vi "LinxUartGetBytesAvailable.vi"(8 "Error In":errorcluster, 10 "Uart Channel":u8, 11 "LINX Resource":T1) -> (0 "Error Out":errorcluster, 1 "Num Bytes":u8, 3 "LINX Resource":T1)   [LabVIEW 2011, in "LMH-LINX.lvlib" / "Local IO.lvlib"]
uses:
  Local IO.lvlib
  Type Defs/LINX Ref.ctl
  Type Defs/Platform.ctl
  Type Defs/Interface.ctl
  Device/Type Defs/LINX Device Config.ctl
  Device/Type Defs/TCP Config.ctl
  Device/Type Defs/Channels.ctl
  Type Defs/Error Type.ctl
  LMH-LINX.lvlib
  Type Defs/Channel FGV States.ctl
  liblinxdevice.dll
  Device/Device.lvlib
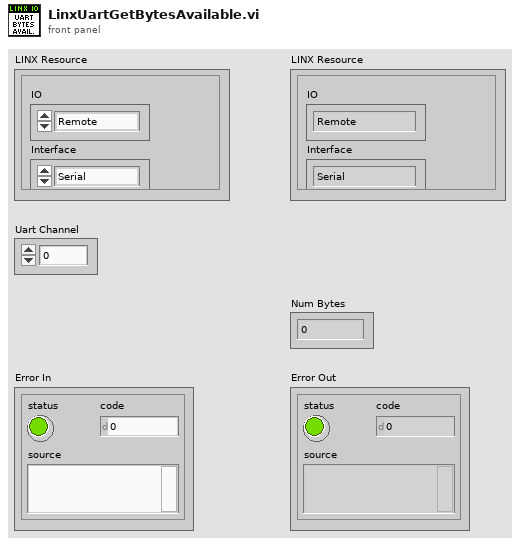
[diagram p1: front panel]
types:
  T1 = typedef "LMH-LINX.lvlib/LINX Ref.ctl" = cluster{"IO":T2, "Interface":T3, "LINX Device Config":T4}
  T2 = typedef "LMH-LINX.lvlib/Platform.ctl" = enum16{"Remote", "Local"}
  T3 = typedef "LMH-LINX.lvlib/Interface.ctl" = enum16{"Serial", "TCP"}
  T4 = typedef "LMH-LINX.lvlib/Device.lvlib/LINX Device Config.ctl" = cluster{"Interface":T3, "COM Port":refnum<visa-resource-name>, "TCP Configuration":T5, "Device Family":u8, "Device ID":u8, "Device Name":string, "TCP Ref":refnum<k5>, "Channels":T6}
  T5 = typedef "LMH-LINX.lvlib/Device.lvlib/TCP Config.ctl" = cluster{"IP Address":string, "Port":u16}
  T6 = typedef "LMH-LINX.lvlib/Channels.ctl" = cluster{"DI":u8[], "DO":u8[], "AI":u8[], "AO":u8[], "PWM":u8[], "QE":u8[], "UART":u8[], "I2C 2":u8[], "SPI":u8[], "CAN":u8[], "Servo":u8[], "AI Ref (V)":dbl, "AI Resolution (Bits)":u8, "AO Ref (V)":dbl, "AO Resolution (Bits)":u8}
  T7 = typedef "LMH-LINX.lvlib/Error Type.ctl" = enum16{"Unknown", "Timeout", "Corrupt Return Packet", "Unable To Connect", "Command Not Supported", "Channel DNE", "Invalid COM Config", "Firmware Version Mismatch", "myRIO Support", "CMD Specific Error", "Local IO Not Supported"}
  T8 = typedef "LMH-LINX.lvlib/Channel FGV States.ctl" = enum16{"Initialize", "Get", "Set"}
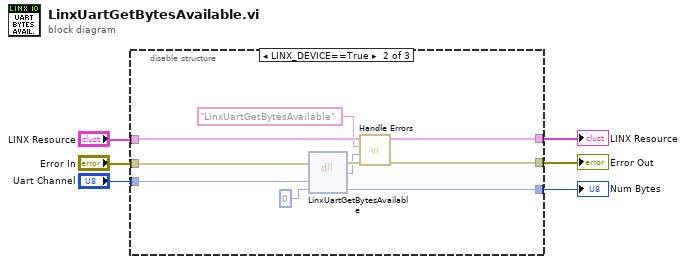
[diagram p0: block diagram]
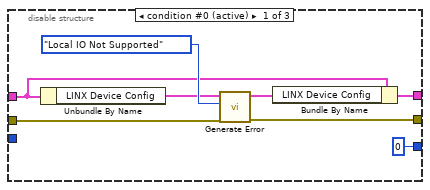
[diagram p2: hidden frame]
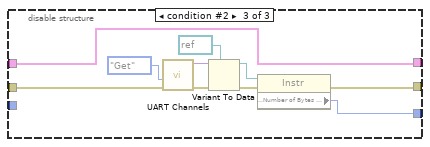
[diagram p3: hidden frame]
diagram:
  n1 = disable-structure shown="LINX_DEVICE==True" {
    disable-tunnel: [w8 w19 w25] -> w5
    disable-tunnel: "LINX Resource" -> [w10 w20 w25]
    disable-tunnel: "Error In" -> [w13 w24 w28]
    disable-tunnel: [w12 w17 w27] -> w6
    disable-tunnel: [u32 0 ("Baud Rate") w22 w26] -> w4
    disable-tunnel: "Uart Channel" -> [_ w23 _]
    frame condition #0 (active) {
      n2 = Unbundle By Name(w10) -> ("LINX Device Config"=w11:T4)
      n3 = call "Generate Error.vi"("Error In"=w13, "Error Type"=Error_Type."Local IO Not Supported", "LINX Device Config"=w11) -> ("Error Out"=w12:errorcluster, "Dup LINX Device Config"=w9:T4)  [unwired: 7 in]
      n4 = Bundle By Name(cluster=w10, "LINX Device Config"=w9) -> (w8:T1)
    }
    frame condition #1 {
      n5 = dll-call lib="liblinxdevice.*" fn="LinxUartGetBytesAvailable"(error in=w24, "channel"=w23, "numBytes"=u8 0) -> (error out=w18:errorcluster, "status"=w15:i32, "numBytes"=w22:u8)  [unwired: 3 in, 1 out]
      n6 = call "Handle Errors.vi"("Error In"=w18, "LinxStatus"=w15, "Function Name"="LinxUartGetBytesAvailable", "LINX Resource"=w20) -> ("Error Out"=w17:errorcluster, "LINX Resource"=w19:T1)  [unwired: 6 in]
    }
    frame condition #2 {
      n7 = call "UART Channels.vi"("Error In"=w28, "Channel State"=Channel_FGV_States."Get") -> ("Error Out"=w29:errorcluster, "UART Channel"=w30:variant)  [unwired: 8 in]
      n8 = Variant To Data(error in=w29, type=refnum<visa-resource-name> refnum ("reference"), Variant=w30) -> (data=w32:refnum<visa-resource-name>, error out=w33:errorcluster)
      n9 = property class="Instr"(reference=w32, error in=w33) -> (error out=w27:errorcluster, "Serial Settings:Number of Bytes at Serial Port"=w26:u32)  [unwired: 1 out]
    }
  }
  "LINX Resource" <- w5
  "Num Bytes" <- w4
  "Error Out" <- w6
